vi "Voltage Dips, Swells, and Interruptions.vi"(0 "one-cycle voltage RMS":T5(array[cluster]), 1 "reset? (F)":bool, 5 "events settings":T4={"swell threshold [%]"=110.0, "dip threshold [%]"=90.0, "interruption threshold [%]"=1.0, "hysteresis [%]"=2.0}, 7 "polyphase only? (F)":bool, 9 "system info in":refnum<class "EP System Info.lvclass">, 11 "error in (no error)":errorcluster) -> (4 "voltage events":T3(array[cluster]), 8 "voltage flags":bool[](array[boolean]), 10 "system info out":refnum<class "EP System Info.lvclass">, 15 "error out":errorcluster)   [LabVIEW 2014, in "NI_EP_Power Quality.lvlib"]
doc: "Detects RMS voltage dips, swells, and interruptions, according to IEC 61000-4-30:2008. EN 50160:2007 defines the default threshold values. You also can specify custom threshold values. You can use EN 50160:2007 to evaluate voltage events that this VI detects.\n\nThis VI supports measuring single-bus single-line or multiple-bus single-line systems."
uses:
  <vilib>/addons/Electrical Power/PQ/NI_EP_Power Quality.lvlib
  <vilib>/addons/Electrical Power/PQ/Common/Controls/ep_Phase.ctl
  <vilib>/addons/Electrical Power/PQ/Common/Controls/ep_Event Type.ctl
  <vilib>/addons/Electrical Power/PQ/Common/Classes/System Info/EP System Info.lvclass
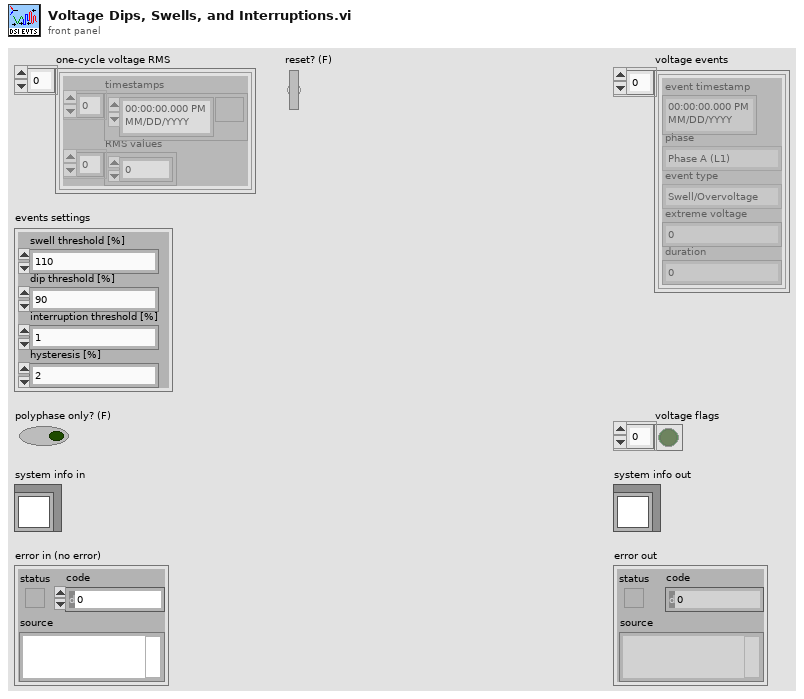
[diagram p1: front panel]
types:
  T1 = typedef "NI_EP_Power Quality.lvlib/ep_Phase.ctl" = enum16{"Phase A (L1)", "Phase B (L2)", "Phase C (L3)", "Phase N", "~3 Phases"}
  T2 = typedef "NI_EP_Power Quality.lvlib/ep_Event Type.ctl" = enum16{"Swell/Overvoltage", "Dip/Undervoltage", "Interruption"}
  T3 = cluster{"event timestamp":timestamp, "phase":T1, "event type":T2, "extreme voltage":dbl, "duration":dbl}[]
  T4 = cluster{"swell threshold [%]":dbl, "dip threshold [%]":dbl, "interruption threshold [%]":dbl, "hysteresis [%]":dbl}
  T5 = cluster{"timestamps":timestamp[], "RMS values":dbl[]}[]
  T6 = cluster{"swell up":dbl, "swell down":dbl, "dip up":dbl, "dip down":dbl, "interrupt up":dbl, "interrupt down":dbl}[]
  T7 = cluster{"event time":timestamp, "phase":T1, "event type":T2, "extreme voltage":dbl, "duration":dbl}[]
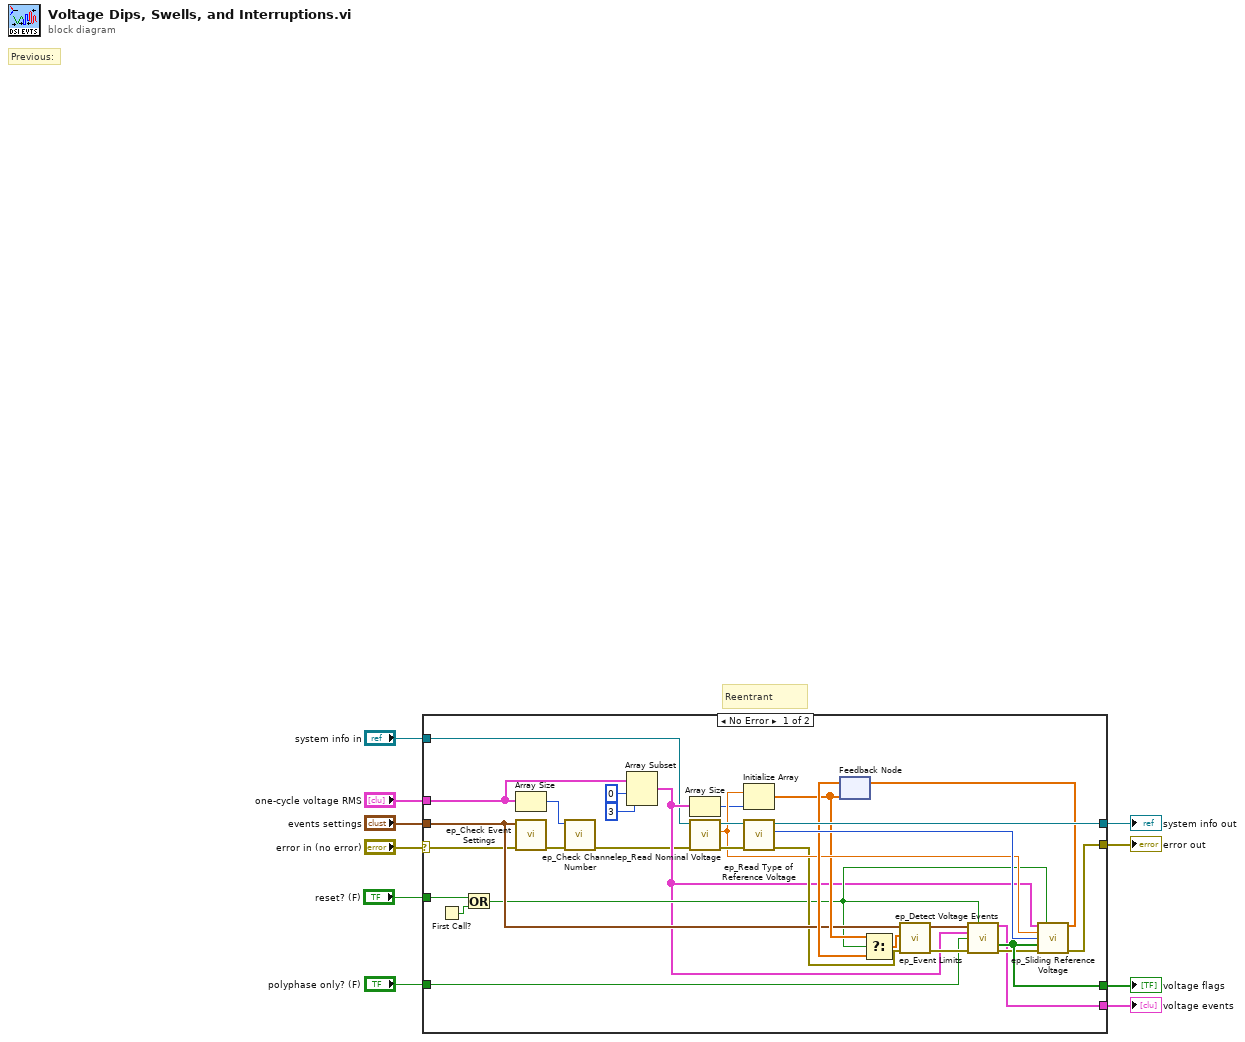
[diagram p0: block diagram]
diagram:
  # "Reentrant"
  # "Previous:"
  n1 = case shown="No Error" "error in (no error)" {
    selector: "error in (no error)" -> [w28 w42]
    tunnel: [w39 w43] -> w10
    tunnel: [w37 _] -> w9
    tunnel: [w13 _] -> w8
    tunnel: "one-cycle voltage RMS" -> [w17 _]
    tunnel: "polyphase only? (F)" -> [w20 _]
    tunnel: [w24 w42] -> w5
    tunnel: "system info in" -> [w14 w43]
    tunnel: "events settings" -> [w31 _]
    tunnel: "reset? (F)" -> [w22 _]
    frame No Error {
      n2 = First Call?() -> (First Call?: T/F=w23:bool)
      n3 = Or(x=w22, y=w23) -> (x .or. y?=w21:bool)
      n4 = Array Size(array=w17) -> (size(s)=w18:i32)
      n5 = call <vilib>:"ep_Check Event Settings.vi"("error in (no error)"=w28, "events settings"=w31) -> ("error out"=w19:errorcluster)  [unwired: 9 in]
      n6 = call <vilib>:"ep_Check Channel Number.vi"("channel number"=w18, "error in (no error)"=w19) -> ("error out"=w15:errorcluster)  [unwired: 13 in]
      n7 = Array Subset(array=w17, index=0, length=3) -> (w16:T5)
      n8 = Array Size(array=w16) -> (size(s)=w33:i32)
      n9 = call <vilib>:"ep_Read Nominal Voltage.vi"("error in (no error)"=w15, "system info in"=w14) -> ("error out"=w40:errorcluster, "nominal voltage [V]"=w35:dbl, "system info out"=w41:refnum<class "EP System Info.lvclass">)  [unwired: 7 in]
      n10 = Initialize Array(w35, w33) -> (w32:dbl[])
      n11 = call <vilib>:"ep_Read Type of Reference Voltage.vi"("error in (no error)"=w40, "system info in"=w41) -> ("error out"=w27:errorcluster, "type of reference voltage"=w38:enum16{"Constant", "Sliding"}, "system info out"=w39:refnum<class "EP System Info.lvclass">)  [unwired: 7 in]
      n12 = feedback #1(w32) -> (w36:dbl[])
      n13 = Select(t=w32, s=w21, f=w36) -> (s? t:f=w29:dbl[])
      n14 = call <vilib>:"ep_Event Limits.vi"("error in (no error)"=w27, "reference voltages"=w29, "events settings"=w31) -> ("error out"=w26:errorcluster, "event limits"=w30:T6)  [unwired: 7 in]
      n15 = call <vilib>:"ep_Detect Voltage Events.vi"("event limits"=w30, "restart (F)"=w21, "voltage RMS (1/2) (1 cycle)"=w16, "polyphase only? (F)"=w20, "error in (no error)"=w26) -> ("voltage events"=w13:T7, "voltage flags"=w37:bool[], "error out"=w25:errorcluster)  [unwired: 8 in]
      n16 = call <vilib>:"ep_Sliding Reference Voltage.vi"("voltage RMS (1/2) (1 cycle)"=w16, "restart (F)"=w21, "nominal voltage [V]"=w35, "type of reference voltage"=w38, "voltage flags"=w37, "error in (no error)"=w25) -> ("reference voltages"=w34:dbl[], "error out"=w24:errorcluster)  [unwired: 8 in]
      n17 = feedback-in #1(w34) -> ()
    }
    frame Error {
    }
  }
  "error out" <- w5
  "voltage events" <- w8
  "voltage flags" <- w9
  "system info out" <- w10
